vi "LabViewPid.vi"() -> ()   [LabVIEW 2018]
uses:
  <vilib>/Platform/TimedLoop/XDataNode/timing_clust.ctl
  <vilib>/Platform/TimedLoop/XDataNode/nitl_modes.ctl
  <vilib>/Platform/TimedLoop/XDataNode/wakeup.ctl
  <vilib>/addons/control/pid/autopid.llb/PID autotuning parameters (FO).ctl
  <vilib>/addons/control/pid/pid.llb/PID (DBL).vi
  <vilib>/platform/TimedLoop/XDataNode/XDataNode.xnode
  <vilib>/Platform/TimedLoop/XDataNode/XDNodeRunTimeDep.lvlib
  <vilib>/addons/control/pid/NI_PID_pid.lvlib
  <vilib>/addons/control/pid/NI_PID_autopid.lvlib
panel:
  out "Tun Delay time (s)":dbl
  out "Tun Time constant (s)":dbl
  out "Tun Process gain":dbl
  out "Tun Td":dbl
  out "Tun Ti":dbl
  out "Tun Kp":dbl
  out "Tunning":bool
  in  "Ring":u16(ring) items=["Off", "Manual", "Automatic", "Tunning"]
  in  "Auto/Manual":bool
  in  "Beta":dbl
  in  "Alfa":dbl
  in  "Type":enum16{"P", "PI", "PID"}(ring)
  in  "Step amplitude":dbl
  in  "Time constant factor":dbl
  in  "Reset Tune":bool
  in  "Delay time (s)":dbl
  in  "Time constant (s)":dbl
  in  "Process gain":dbl
  out "Tunning Complete":bool
  out "dt PID":dbl
  in  "Reset PID":bool
  out "dt loop":dbl
  out "Loop and out":errorcluster
  in  "Frequency":dbl(slide) scale=1.0..100.0
  out "Interval":i64
  in  "Stop":bool
  out "Counter":i32
  in  "Manual":dbl(slide) scale=0.0..255.0
  in  "Setpoint 3":dbl(slide) scale=0.0..255.0
  out "Setpoint":sgl(knob) scale=0.0..300.0
  out "Temperature":sgl(slide) scale=0.0..300.0
  out "Manual":i16(knob) scale=0.0..255.0
  out "Output":i16(knob) scale=0.0..255.0
  out "Off Hook":bool
  out "Communication Failure":bool
  out "Updating":bool
  in  "Format":string(combo)
  in  "Delimiter":string(combo)
  out "Canceled":bool
  out "Logging to file":bool
  out "File":errorcluster
  out "Time (ms)":u32
  out "Single Update (Multiple Plots, stacked)":cluster{"Temperature":sgl, "Setpoint":sgl, sgl}(graph)
  out "Kd":sgl
  out "Ki":sgl
  in  "Set Kp":sgl
  in  "Set Td":sgl
  in  "Set Ti":sgl
  in  "file path (use dialog)":path
  in  "disable buffering (F)":bool
  in  "Start/stop file":bool
  in  "Apply Max time":bool
  in  "Scale":bool
  in  "Max time":dbl
  out "Modbus":errorcluster
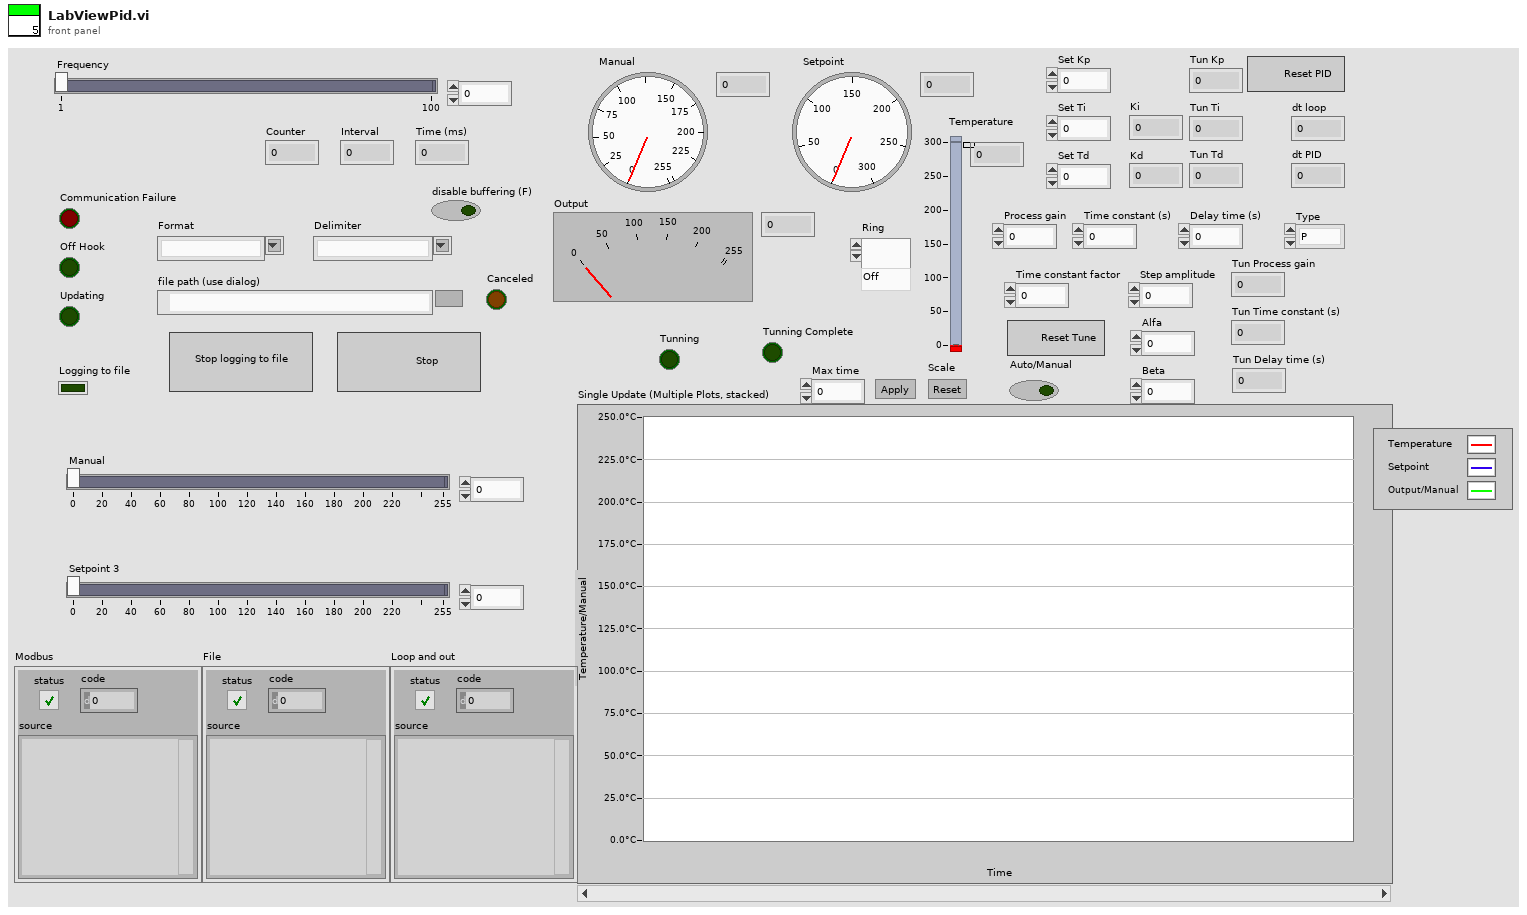
[diagram p1: front panel]
types:
  T1 = cluster{"process gain":dbl, "time constant (s)":dbl, "delay time (s)":dbl}
  T2 = cluster{"proportional gain (Kc)":dbl, "integral time (Ti, min)":dbl, "derivative time (Td, min)":dbl}
  T3 = typedef "NI_PID_autopid.lvlib/PID autotuning parameters (FO).ctl" = cluster{"type of controller":u16, "time constant factor":dbl, "step amplitude":dbl}
  T4 = enum16{"open", "replace", "create", "open or create", "replace or create", "replace or create with confirmation"}
  T5 = typedef "XDNodeRunTimeDep.lvlib/timing_clust.ctl" = cluster{"Expected End [f-1]":u64, "Actual End [f-1]":u64, "Finished Late? [f-1]":bool, "Expected End [i-1]":u64, "Actual End [i-1]":u64, "Finished Late? [i-1]":bool, "Expected Start [i]":u64, "Actual Start [i]":u64, "Expected Start [f]":u64, "Actual Start [f]":u64, "Source Name":string, "Structure Name":string, "Period":i64, "Deadline":i64, "Offset":i64, "Start":i64, "Priority":i32, "Timeout":i32, "Mode":T6, "Wakeup Reason":T7, "Error":errorcluster, "Source Type":string, "Secondary Source Type":string, "Global End Time":u64, "Global Start Time":u64, "Frame Duration":u64, "Iteration Duration":u64, "Assigned CPU":i32, "I/O Scan Engine Mode":u32}
  T6 = typedef "XDNodeRunTimeDep.lvlib/nitl_modes.ctl" = enum32{"No Change", "Process missed periods, maintain original phase", "Discard missed periods, maintain original phase", "Process missed periods, ignore original phase", "Discard missed periods, ignore original phase"}
  T7 = typedef "XDNodeRunTimeDep.lvlib/wakeup.ctl" = enum32{"Normal", "Aborted", "Asynchronous wakeup", "Timing source error", "Timed loop error", "Timeout"}
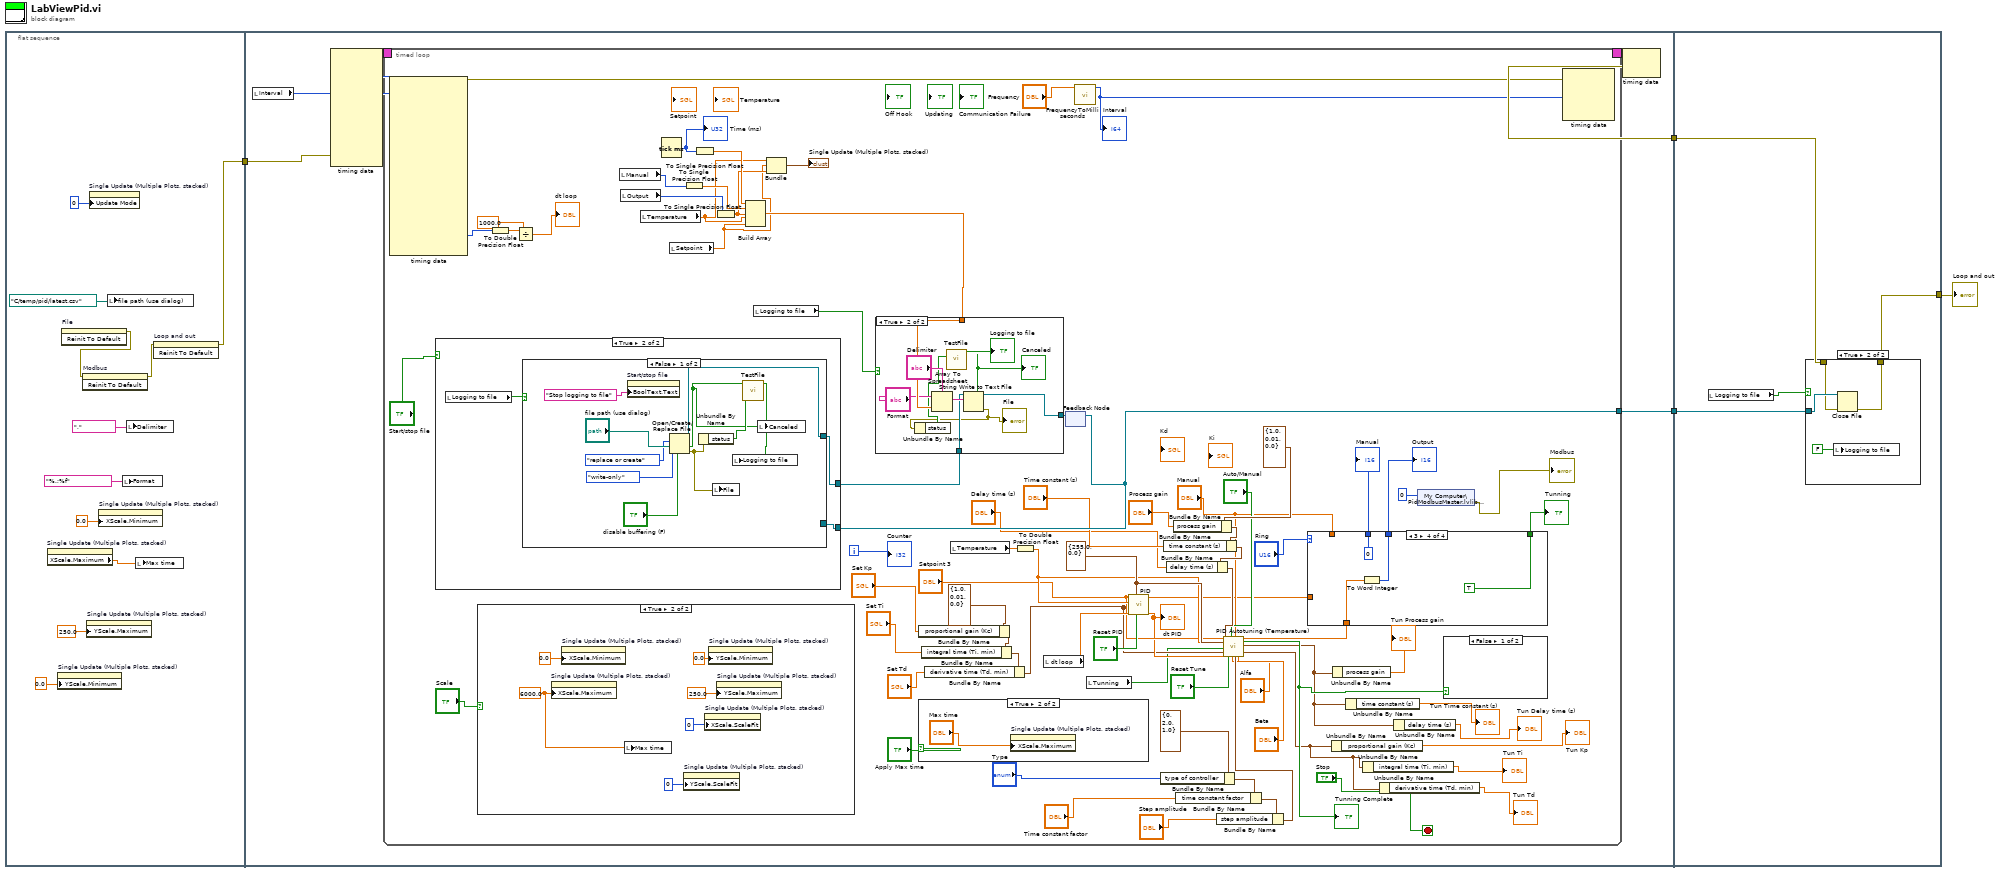
[diagram p0: block diagram]
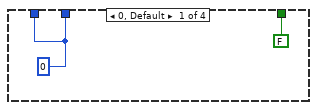
[diagram p3: hidden frame]
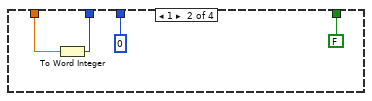
[diagram p4: hidden frame]
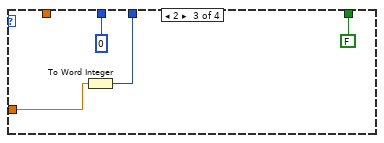
[diagram p5: hidden frame]
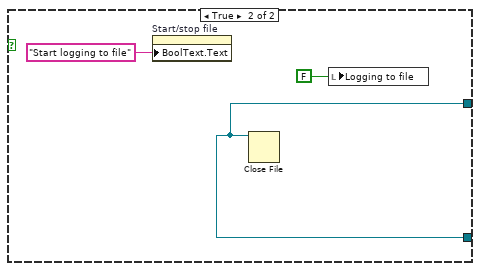
[diagram p9: hidden frame]
diagram:
  n1 = flat-sequence {
    tunnel: [w5] -> w4
    tunnel: [w18] -> w3
    tunnel: [w17] -> w2
    tunnel: w4 -> [w16]
    tunnel: w3 -> [w162]
    tunnel: w2 -> [w163]
    tunnel: [w161] -> w1
    frame #0 {
      n2 = property on="Single Update (Multiple Plots, stacked)" class="WFChart (strict)"() -> ("XScale.Maximum"=w11:dbl)  [unwired: 2 in, 2 out]
      n3 = property on="Single Update (Multiple Plots, stacked)" class="WFChart (strict)"("YScale.Minimum"=0.0 ("Y Scale.Range:Minimum")) -> ()  [unwired: 2 in, 2 out]
      n4 = invoke on="File" class="Clust (strict)" method="Reinit To Default"() -> (error out=w7:errorcluster)  [unwired: 3 in, 2 out]
      n5 = invoke on="Modbus" class="Clust (strict)" method="Reinit To Default"(error in=w7) -> (error out=w6:errorcluster)  [unwired: 2 in, 2 out]
      n6 = property on="Single Update (Multiple Plots, stacked)" class="WFChart (strict)"("YScale.Maximum"=250.0 ("Y Scale.Range:Maximum")) -> ()  [unwired: 2 in, 2 out]
      n7 = property on="Single Update (Multiple Plots, stacked)" class="WFChart (strict)"("Update Mode"=u8 0) -> ()  [unwired: 2 in, 2 out]
      n8 = property on="Single Update (Multiple Plots, stacked)" class="WFChart (strict)"("XScale.Minimum"=0.0 ("X Scale.Range:Minimum")) -> ()  [unwired: 2 in, 2 out]
      n9 = local write "file path (use dialog)"(path "C:/temp/pid/latest.csv" ("file path (use dialog)")) -> ()
      n10 = local write "Format"("%.;%f" ("Format")) -> ()
      n11 = local write "Delimiter"("," ("Delimiter")) -> ()
      n12 = local write "Max time"(w11) -> ()
      n13 = invoke on="Loop and out" class="Clust (strict)" method="Reinit To Default"(error in=w6) -> (error out=w5:errorcluster)  [unwired: 2 in, 2 out]
    }
    frame #1 {
      n14 = local read "Interval"() -> (w19:i64)
      n15 = node-c288(w19, w16) -> (w21:T5)  [unwired: 8 in]
      n16 = timed-loop {
        timing: w21 -> [_]
        timing-out: [_] -> w20
        tunnel: [w86] -> w17
        i -> [w96]
        stop <- "Stop" stop-if-true
        w70 = cluster{"output high":dbl, "output low":dbl} {"output high"=255.0, "output low"=0.0} ("output range")
        n17 = node-c288() -> (w78:errorcluster, w76:i64)  [unwired: 1 in, 15 out]
        n18 = case shown="True" "Scale" {
          frame False {
          }
          frame True {
            w116 = 6000.0 ("X Scale.Range:Maximum")
            n19 = property on="Single Update (Multiple Plots, stacked)" class="WFChart (strict)"("XScale.Maximum"=w116) -> ()  [unwired: 2 in, 2 out]
            n20 = property on="Single Update (Multiple Plots, stacked)" class="WFChart (strict)"("XScale.Minimum"=0.0 ("X Scale.Range:Minimum")) -> ()  [unwired: 2 in, 2 out]
            n21 = local write "Max time"(w116) -> ()
            n22 = property on="Single Update (Multiple Plots, stacked)" class="WFChart (strict)"("YScale.ScaleFit"=u8 0 ("Y Scale.Scale Fit")) -> ()  [unwired: 2 in, 2 out]
            n23 = property on="Single Update (Multiple Plots, stacked)" class="WFChart (strict)"("XScale.ScaleFit"=u8 0 ("X Scale.Scale Fit")) -> ()  [unwired: 2 in, 2 out]
            n24 = property on="Single Update (Multiple Plots, stacked)" class="WFChart (strict)"("YScale.Minimum"=0.0 ("Y Scale.Range:Minimum")) -> ()  [unwired: 2 in, 2 out]
            n25 = property on="Single Update (Multiple Plots, stacked)" class="WFChart (strict)"("YScale.Maximum"=250.0 ("Y Scale.Range:Maximum")) -> ()  [unwired: 2 in, 2 out]
          }
        }
        n26 = To Double Precision Float(number=w76) -> (double precision float=w75:dbl)
        n27 = Divide(x=w75, y=1000.0) -> (x/y=→"dt loop":dbl)
        n28 = local read "Manual"() -> (w90:i16)
        n29 = local read "Output"() -> (w91:i16)
        n30 = local read "Temperature"() -> (w84:sgl)
        n31 = Tick Count (ms)() -> (millisecond timer value=w93:u32)
        "Time (ms)" <- w93
        n32 = local read "Setpoint"() -> (w82:sgl)
        n33 = To Single Precision Float(number=w90) -> (single precision float=w92:sgl)
        n34 = To Single Precision Float(number=w93) -> (single precision float=w94:sgl)
        n35 = To Single Precision Float(number=w91) -> (single precision float=w83:sgl)
        n36 = Build Array(w94, w92, w83, w84, w82) -> (w95:sgl[])
        n37 = local read "Logging to file"() -> (w85:bool)
        n38 = Bundle("Temperature"=w84, "Setpoint"=w82, w83) -> (→"Single Update (Multiple Plots, stacked)":cluster{"Temperature":sgl, "Setpoint":sgl, sgl})  [unwired: 1 in]
        n39 = Bundle By Name(cluster=T2 {"proportional gain (Kc)"=1.0, "integral time (Ti, min)"=0.01, "derivative time (Td, min)"=0.0} ("PID gains out"), "proportional gain (Kc)"="Set Kp") -> (w65:T2)
        n40 = case shown="True" "Apply Max time" {
          frame False {
          }
          frame True {
            n41 = property on="Single Update (Multiple Plots, stacked)" class="WFChart (strict)"("XScale.Maximum"="Max time") -> ()  [unwired: 2 in, 2 out]
          }
        }
        n42 = Bundle By Name(cluster=w65, "integral time (Ti, min)"="Set Ti") -> (w64:T2)
        n43 = Bundle By Name(cluster=w64, "derivative time (Td, min)"="Set Td") -> (w53:T2)
        n44 = local read "Temperature"() -> (w69:sgl)
        n45 = To Double Precision Float(number=w69) -> (double precision float=w68:dbl)
        n46 = local read "dt loop"() -> (w72:dbl)
        n47 = feedback #1() -> (w86:refnum<file>)  [unwired: 1 in]
        n48 = case shown="True" "Start/stop file" {
          tunnel: [w120 w122] -> w89
          tunnel: w86 -> [w120 w121]
          frame False {
          }
          frame True {
            n49 = local read "Logging to file"() -> (w123:bool)
            n50 = case shown="False" w123 {
              tunnel: [w127 w135] -> w122
              tunnel: w121 -> [_ w135]
              frame False {
                n51 = property on="Start/stop file" class="Bool"("BoolText.Text"="Stop logging to file" ("Boolean Text.Text")) -> ()  [unwired: 2 in, 2 out]
                n52 = Open/Create/Replace File(file path (use dialog)="file path (use dialog)", operation (0:open)=T4."replace or create", access (0:read/write)=enum16{"read/write", "read-only", "write-only"}."write-only", disable buffering (F)="disable buffering (F)") -> (refnum out=w127:refnum<file>, cancelled=w128:bool, error out=w124:errorcluster)  [unwired: 2 in]
                n53 = Unbundle By Name(w124) -> ("status"=w129:bool)
                n54 = local write "File"(w124) -> ()
                n55 = call "TestFile.vi"("status"=w129, "cancelled"=w128) -> ("IsOpen"=w130:bool)  [unwired: 9 in]
                n56 = local write "Logging to file"(w130) -> ()
                n57 = local write "Canceled"(w128) -> ()
              }
              frame True {
                n58 = property on="Start/stop file" class="Bool"("BoolText.Text"="Start logging to file" ("Boolean Text.Text")) -> ()  [unwired: 2 in, 2 out]
                n59 = Close File(refnum=w135) -> ()  [unwired: 1 in, 2 out]
                n60 = local write "Logging to file"(FALSE ("Logging to file")) -> ()
              }
            }
          }
        }
        n61 = case shown="True" w85 {
          tunnel: w95 -> [_ w147]
          tunnel: [w137 w144] -> w87
          tunnel: w89 -> [w137 w142]
          frame False {
          }
          frame True {
            n62 = Array To Spreadsheet String(delimiter (Tab)="Delimiter", array=w147, 3:"Format") -> (spreadsheet string=w143:string)
            n63 = Write to Text File(file (use dialog)=w142, text=w143) -> (refnum out=w144:refnum<file>, cancelled=w140:bool, error out=w138:errorcluster)  [unwired: 2 in]
            "Canceled" <- w140
            "File" <- w138
            n64 = Unbundle By Name(w138) -> ("status"=w139:bool)
            n65 = call "TestFile.vi"("status"=w139, "cancelled"=w140) -> ("IsOpen"=→"Logging to file":bool)  [unwired: 9 in]
          }
        }
        n66 = feedback-in #1(w87) -> ()
        n67 = call "FrequencyToMilliseconds.vi"("Frequency"="Frequency") -> ("Numeric"=w97:i64)  [unwired: 10 in]
        "Interval" <- w97
        n68 = local read "Tunning"() -> (w34:bool)
        n69 = call-poly <vilib>:"PID.vi"("reinitialize? (F)"="Reset PID", "output range"=w70, "dt (s)"=w72, "PID gains"=w53, "process variable"=w68, "setpoint"="Setpoint 3") -> ("dt out (s)"=w66:dbl, "output"=w37:dbl)  [unwired: 4 in]
        "dt PID" <- w66
        n70 = Bundle By Name(cluster=T3 {"type of controller"=0, "time constant factor"=2.0, "step amplitude"=1.0} ("autotuning parameters"), "type of controller"="Type") -> (w49:T3)
        n71 = Bundle By Name(cluster=T1 {"process gain"=1.0, "time constant (s)"=0.01, "delay time (s)"=0.0} ("plant parameters in"), "process gain"="Process gain") -> (w57:T1)
        n72 = Bundle By Name(cluster=w57, "time constant (s)"="Time constant (s)") -> (w56:T1)
        n73 = Bundle By Name(cluster=w56, "delay time (s)"="Delay time (s)") -> (w51:T1)
        n74 = Bundle By Name(cluster=w49, "time constant factor"="Time constant factor") -> (w48:T3)
        n75 = Bundle By Name(cluster=w48, "step amplitude"="Step amplitude") -> (w47:T3)
        n76 = call <vilib>:"PID Autotuning (Temperature).vi"("desired temperature"="Setpoint 3", "measured temperature"=w68, "plant parameters in"=w51, "autotune? (F)"=w34, "PID gains in"=w53, "dt (s)"=w66, "output range"=w70, "reinitialize? (F)"="Reset Tune", "auto? (T)"="Auto/Manual", "beta"="Beta", "manual control"="Manual", "autotuning parameters"=w47, "alpha"="Alfa") -> ("output"=w36:dbl, "tuning completed?"=w33:bool, "plant parameters out"=w32:T1, "PID gains out"=w31:T2)  [unwired: 3 in]
        "Tunning Complete" <- w33
        n77 = case shown="3" "Ring" {
          tunnel: "Manual" -> [_ w104 _ _]
          tunnel: w37 -> [_ _ w108 _]
          tunnel: w36 -> [_ _ _ w112]
          tunnel: [FALSE FALSE FALSE TRUE] -> w35
          tunnel: [w99 i16 0 w106 w110] -> w24
          tunnel: [w99 w102 i16 0 i16 0] -> w23
          frame 0, Default {
            w99 = i16 0
          }
          frame 1 {
            n78 = To Word Integer(number=w104) -> (16bit integer=w102:i16)
          }
          frame 2 {
            n79 = To Word Integer(number=w108) -> (16bit integer=w106:i16)
          }
          frame 3 {
            n80 = To Word Integer(number=w112) -> (16bit integer=w110:i16)
          }
        }
        "Tunning" <- w35
        "Output" <- w24
        "Manual" <- w23
        n81 = Unbundle By Name(w31) -> ("proportional gain (Kc)"=→"Tun Kp":dbl)
        n82 = Unbundle By Name(w32) -> ("process gain"=→"Tun Process gain":dbl)
        n83 = Unbundle By Name(w32) -> ("time constant (s)"=→"Tun Time constant (s)":dbl)
        n84 = Unbundle By Name(w31) -> ("integral time (Ti, min)"=→"Tun Ti":dbl)
        n85 = Unbundle By Name(w31) -> ("derivative time (Td, min)"=→"Tun Td":dbl)
        n86 = Unbundle By Name(w32) -> ("delay time (s)"=→"Tun Delay time (s)":dbl)
        n87 = shared-variable "My Computer\\PidModbusMaster.lvlib\\S400001"(i16 0 ("S400001")) -> (error out=→"Modbus":errorcluster)  [unwired: 1 in]
        n88 = case shown="False" w33 {
          frame False {
          }
          frame True {
          }
        }
        n89 = node-c288(w78, w97) -> ()  [unwired: 2 in, 1 out]
        "Counter" <- w96
      }
      n90 = node-c288(w20) -> (w18:errorcluster)
    }
    frame #2 {
      n91 = local read "Logging to file"() -> (w164:bool)
      n92 = case shown="True" w164 {
        tunnel: w163 -> [_ w169]
        tunnel: w162 -> [w165 w168]
        tunnel: [w165 w167] -> w161
        frame False {
        }
        frame True {
          n93 = local write "Logging to file"(FALSE ("Logging to file")) -> ()
          n94 = Close File(refnum=w169, error in=w168) -> (error out=w167:errorcluster)  [unwired: 1 out]
        }
      }
    }
  }
  "Loop and out" <- w1
